vi "AddTestSuite_NoParent_TagNameIncludesPrefixAndName.vi"() -> (0 "error out":errorcluster)   [LabVIEW 2019, in "ResultTreeTest.lvlib"]
uses:
  ResultTreeTest.lvlib
  2a6c7ef5-d8ea-4de4-ba7d-c6663dbf2225.vi
  Constraint/IsEqual/Create.vi
  Constraint/IsEqual/IsEqual.lvclass
  ResultTree/ResultTree.lvclass
panel:
  in  "Tree":string(tree)
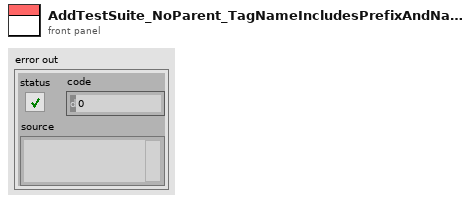
[diagram p1: front panel]
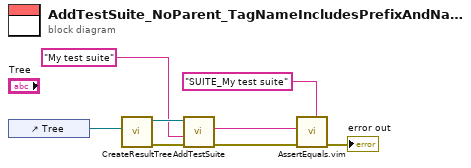
[diagram p0: block diagram]
diagram:
  n1 = control-ref of="Tree"() -> (w7:refnum<vi>)
  n2 = call "CreateResultTree.vi"("Tree Refnum"=w7) -> ("error out"=w6:errorcluster, "ResultTree out"=w5:refnum<class "ResultTree.lvclass">)  [unwired: 9 in]
  n3 = call "AddTestSuite.vi"("error in (no error)"=w6, "Name"="My test suite", "ResultTree in"=w5) -> ("error out"=w3:errorcluster, "Tag Name"=w2:string)  [unwired: 6 in, 1 out]
  n4 = call "AssertEquals.vim"("Expected"="SUITE_My test suite", "error in (no error)"=w3, "Actual"=w2) -> ("error out"=→"error out":errorcluster)  [unwired: 8 in]
